vi "main002.vi"() -> ()   [LabVIEW 2018]
uses:
  subvi/Newport ESP301/Newport ESP301.lvlib
  <userlib>/caLab/Private/Put_DBL_PV.vi
  <userlib>/caLab/Private/Put_I32-1D_PV-1D.vi
  <userlib>/caLab/Private/Put_I32_PV.vi
  <userlib>/caLab/Private/Get_PV.vi
  <vilib>/DAQmx/write.llb/DAQmx Write (Analog DBL 1Chan 1Samp).vi
  <vilib>/DAQmx/create/channels.llb/DAQmx Create Channel (AO-Voltage-Basic).vi
  700a36db-ce49-4288-8972-970908bb0277.vi
  c1e43a28-daf4-4db5-b676-cc48828ec5f1.vi
panel:
  out "Intensity Graph":dbl[][](graph)
  in  "Tab Control":enum32{"Control", "Automation", "Configuration"}(tab)
  in  "delay_go":bool
  in  "delay_destination_fs":dbl=0.1 caption="Destination [fs]"
  in  "delay_destination_mm":dbl=0.1 caption="Destination [mm]"
  in  "delay_velocity":dbl=0.1 caption="velocity [mm/s]"
  in  "set_vel":bool
  in  "time_zero":dbl=1.0 caption="t0 [mm]"
  out "delay_pos_mm":dbl=1.0624 caption="Position [mm]"
  out "delay_pos_fs":dbl=416.2879908072938 caption="Time [fs]"
  in  "delay_set_t0":bool
  in  "delay_rel_mm_+":bool
  in  "delay_rel_mm_-":bool
  in  "delay_stepsize_mm":dbl=1.0 caption="step size [mm]"
  in  "delay_stepsize_fs":dbl=1.0 caption="step size [fs]"
  in  "delay_rel_fs_+":bool
  in  "delay_rel_fs_-":bool
  in  "pump_rel_+":bool
  in  "pump_rel_-":bool
  in  "pump_rel_delta":dbl=1.0 caption="step size [deg]"
  out "pump_position":dbl=1.0624 caption="Position [deg]"
  in  "probe_rel_+":bool
  in  "probe_rel_-":bool
  in  "probe_rel_delta":dbl=1.0 caption="step size [deg]"
  out "probe_position":dbl=416.2879908072938 caption="Position [deg]"
  in  "delay_mode_select":enum32{"Discrete Mode", "Continous Mode"}(tab)
  in  "delay_waypoints":string[][](table)
  in  "delay_waypoint_mode":bool=TRUE
  in  "acquisition time [ms]":u32=1000
  in  "delay_speedpoints":string[][](table)
  in  "start":bool
  in  "stop":bool
  in  "pump_waypoints":string[][](table)
  in  "pump_waypoint_mode":bool=TRUE
  in  "probe_waypoints":string[][](table)
  in  "probe_waypoint_mode":bool=TRUE
  in  "pump_offset":dbl=1.0
  in  "probe_offset":dbl=1.0
  in  "pump_set_offset":bool
  in  "probe_set_offset":bool
  in  "ESP Patch":u32[](array[numeric]) min=1 max=3 step=1
  in  "ESP301 COM PORT":refnum<visa-resource-name>="COM8"
  in  "Serial Link (RS232)":enum16{"RS232", "USB"}(ring)=enum."USB"
  in  "DAC physical channel":tag="Dev3/ao1"
  out "ESP error":errorcluster
  out "DAC error":errorcluster
  out "DAC_Voutput":dbl=5.25341140860948 caption="output voltage"
  in  "pvname_delay":string="caLabTest:DELAY"
  in  "pvname_pumprot":string="caLabTest:DELAY"
  in  "pvname_proberot":string="caLabTest:DELAY"
  in  "main_close":bool
  # "lambda / 2"
  # "Delay"
  # "lambda / 4"
  # "delaystage"
  # "stage will scan back and forth for each pump / probe angle"
  # "Pump Waveplate"
  # "Probe Waveplate"
  # "Delaystage"
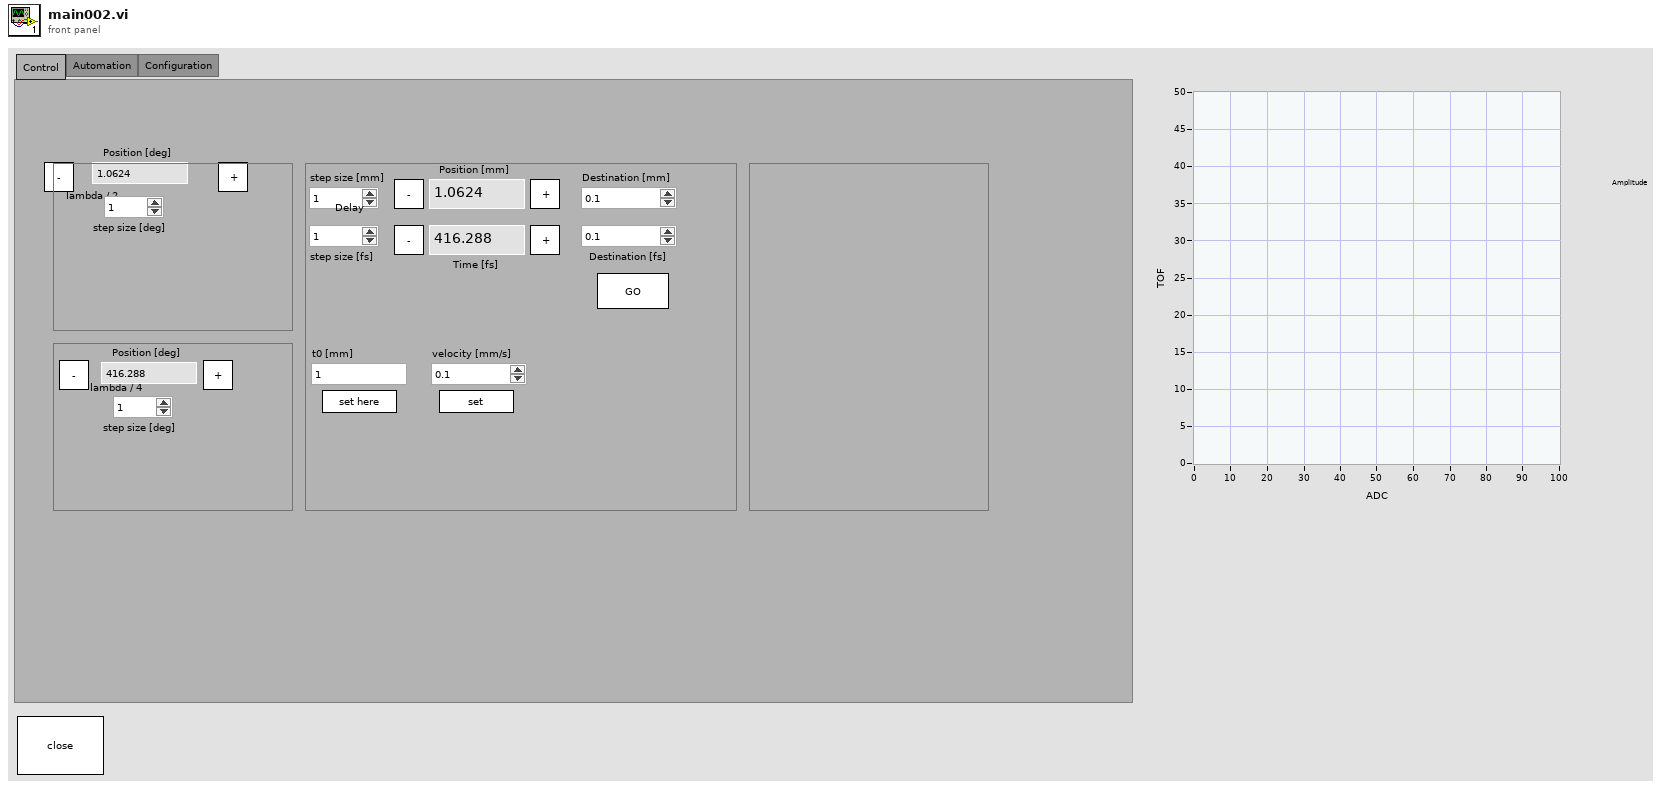
[diagram p1: front panel]
types:
  T1 = cluster{"Field Name":string, "Field Value":string}[]
  T2 = cluster{"dev1_cmd":refnum<queue>, "dev2_cmd":refnum<queue>, "meas_cmd":refnum<queue>}
  T3 = cluster{"dev1_data":refnum<queue>, "dev2_data":refnum<queue>}
  T4 = cluster{"pvname_pumprot":string, "Data Type":string, "Fields":cluster{"Field Name":string, "Field Value":string}[]}
  T5 = cluster{"pvname_delay":string, "Data Type":string, "Fields":cluster{"Field Name":string, "Field Value":string}[]}
  T6 = cluster{"pvname_proberot":string, "Data Type":string, "Fields":cluster{"Field Name":string, "Field Value":string}[]}
  T7 = cluster{"pvname_proberot":string, "Data Type":string, "Fields":cluster{"Field Name":string, "Field Value":string}[]}[]
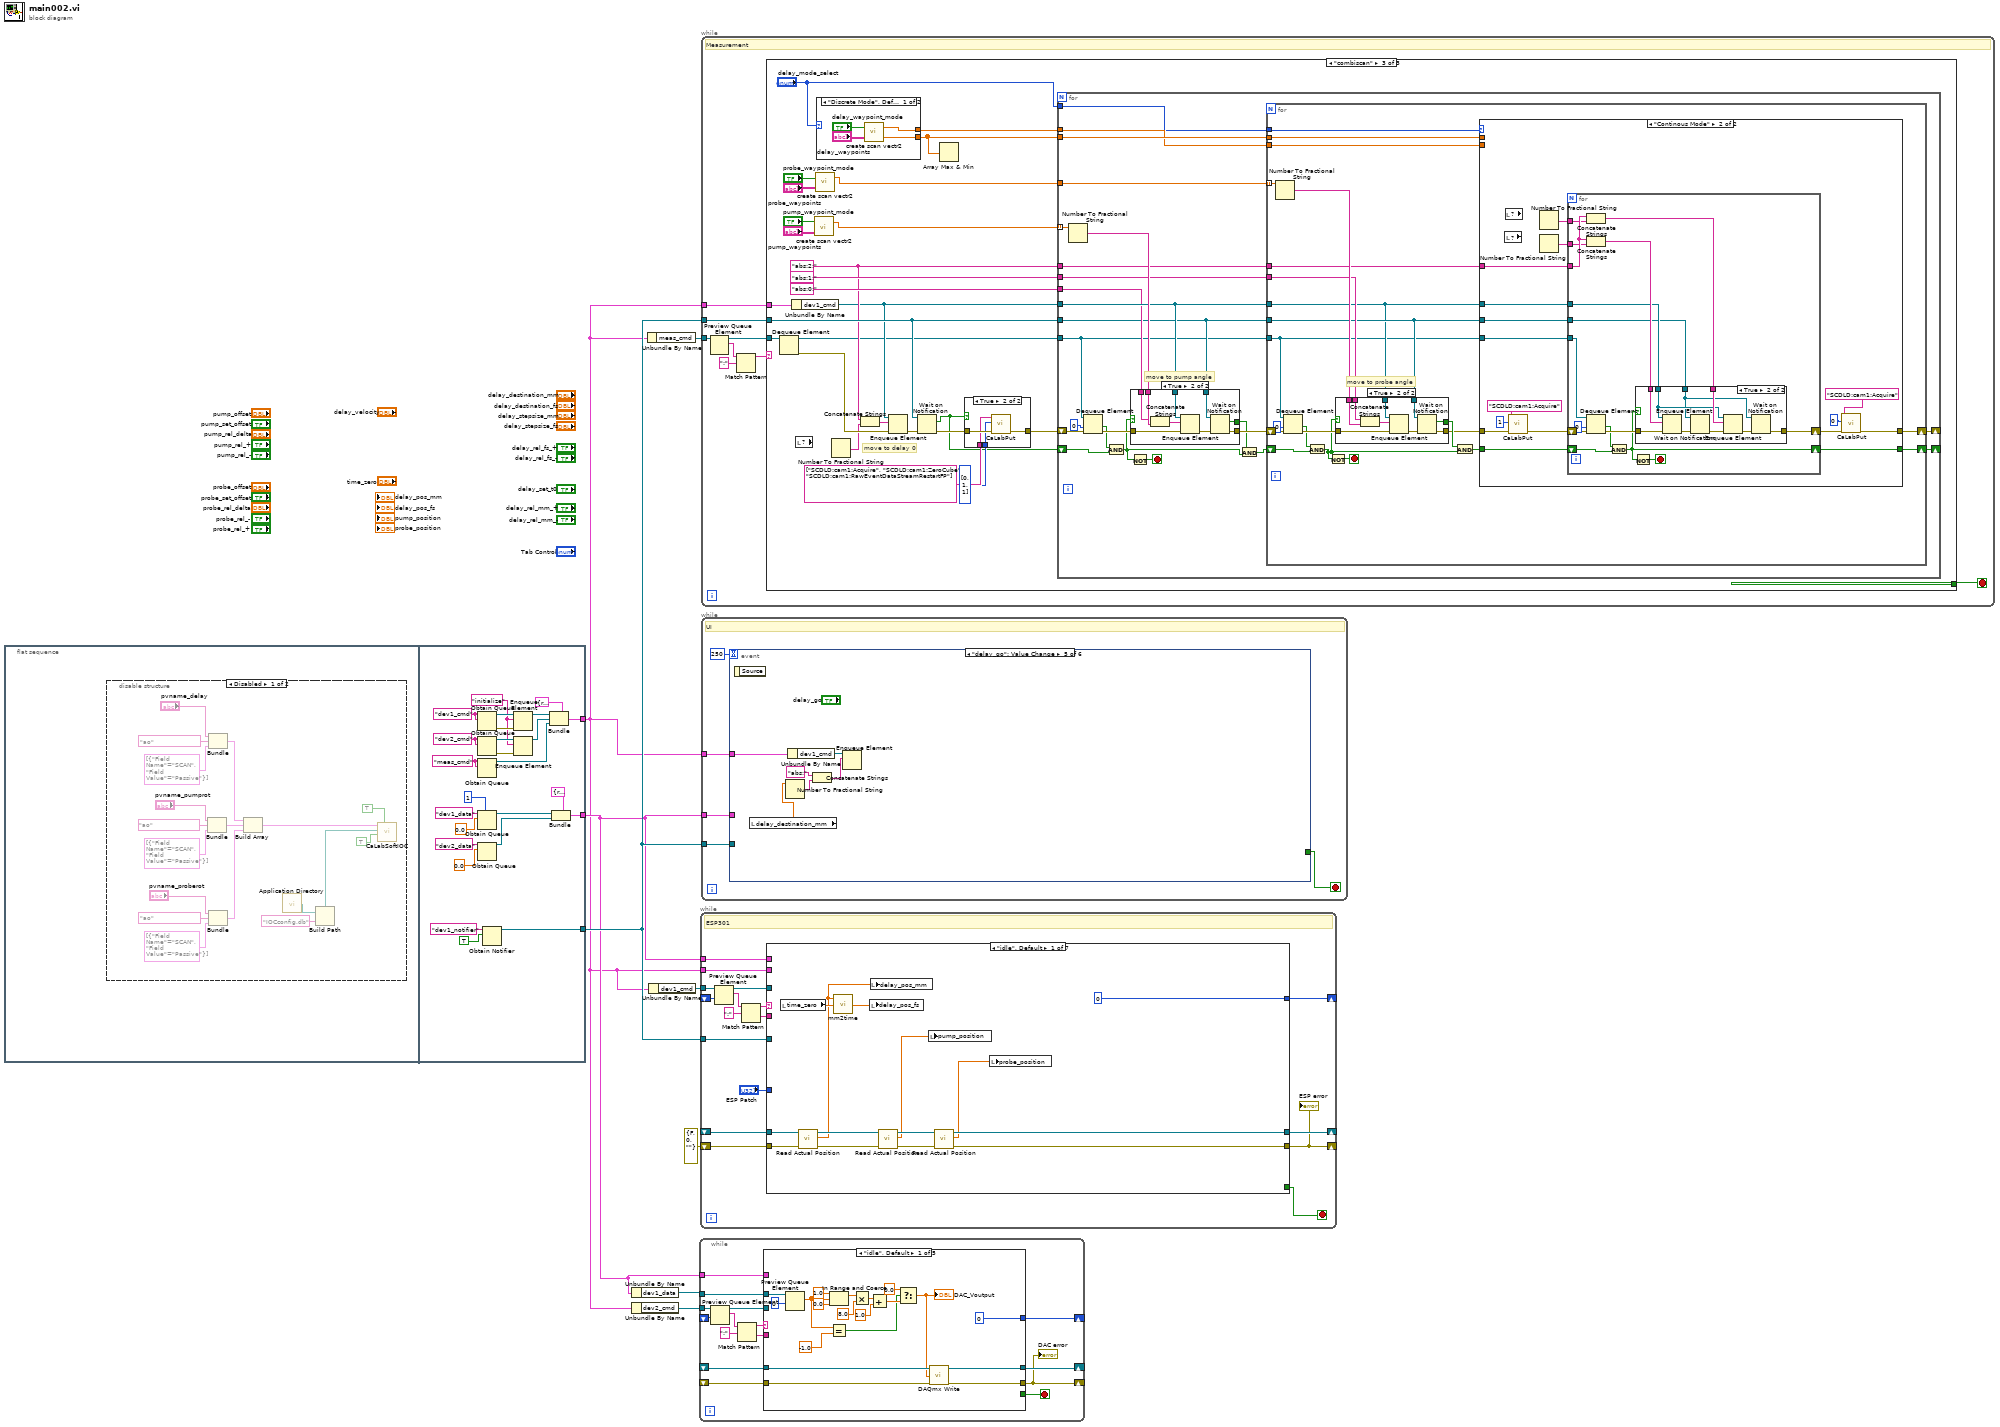
[diagram p0: block diagram]
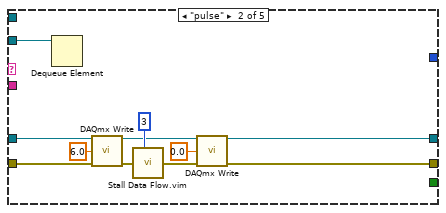
[diagram p2: hidden frame]
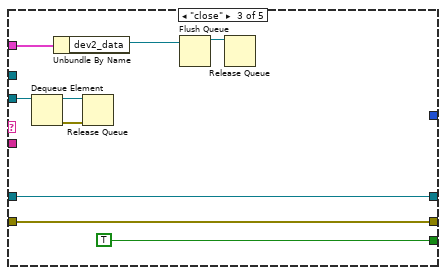
[diagram p3: hidden frame]
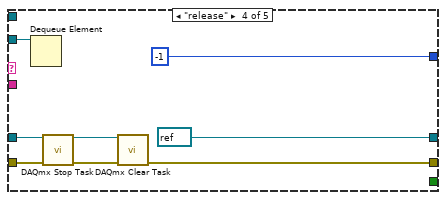
[diagram p4: hidden frame]
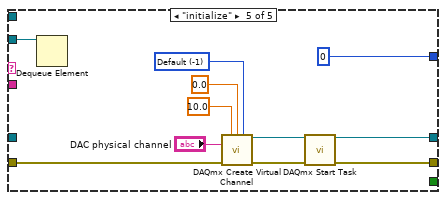
[diagram p5: hidden frame]
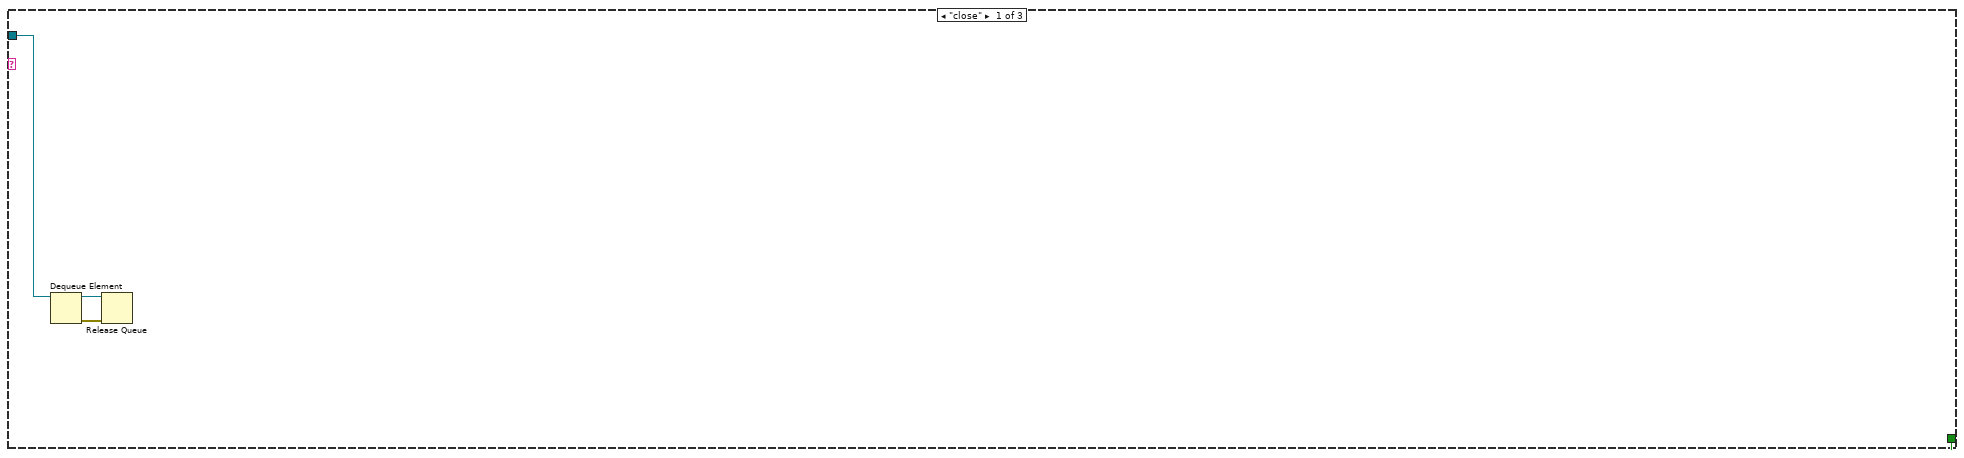
[diagram p7: hidden frame]
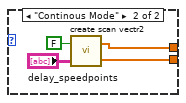
[diagram p9: hidden frame]
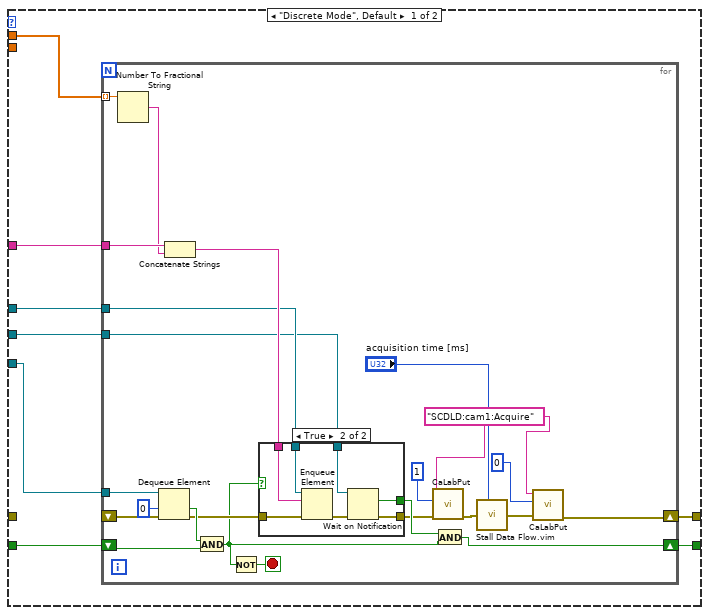
[diagram p12: hidden frame]
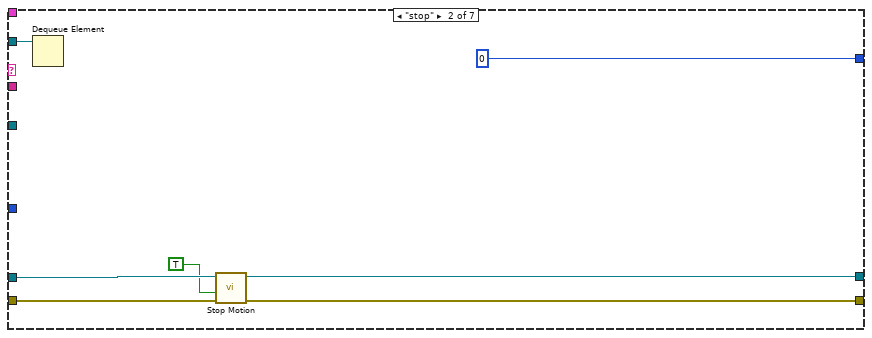
[diagram p16: hidden frame]
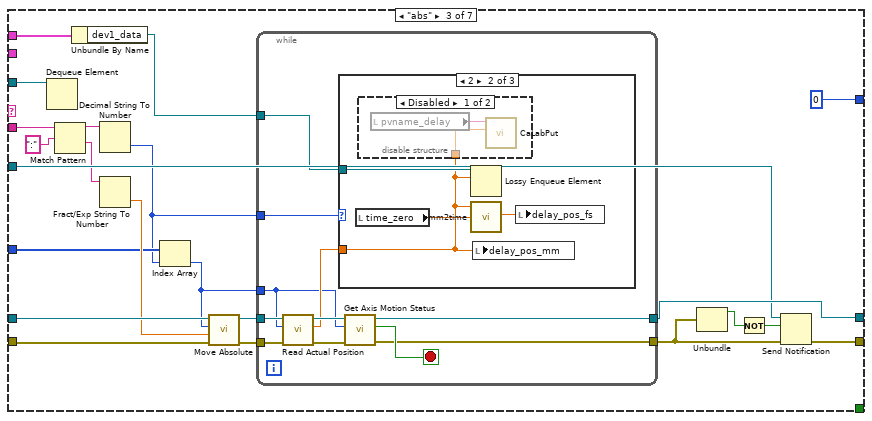
[diagram p17: hidden frame]
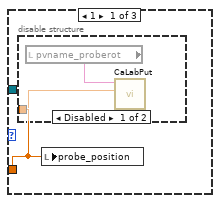
[diagram p18: hidden frame]
diagram:
  n1 = flat-sequence {
    tunnel: [w33] -> w2
    tunnel: [w28] -> w5
    tunnel: [w27] -> w1
    frame #0 {
      n2 = disable-structure shown="Disabled" {
        frame Disabled {
          n3 = Bundle("pvname_pumprot"="pvname_pumprot", "Data Type"="ao", "Fields"=T1 [{"Field Name"="SCAN", "Field Value"="Passive"}]) -> (w11:T4)  [unwired: 1 in]
          n4 = Bundle("pvname_delay"="pvname_delay", "Data Type"="ao", "Fields"=T1 [{"Field Name"="SCAN", "Field Value"="Passive"}]) -> (w18:T5)  [unwired: 1 in]
          n5 = Bundle("pvname_proberot"="pvname_proberot", "Data Type"="ao", "Fields"=T1 [{"Field Name"="SCAN", "Field Value"="Passive"}]) -> (w10:T6)  [unwired: 1 in]
          n6 = Build Array(w18, w11, w10) -> (w9:T7)
          n7 = call <vilib>:"Application Directory.vi"() -> ("Application Directory"=w25:path)
          n8 = Build Path(base path=w25, name or relative path="IOCconfig.db") -> (appended path=w26:path)
          n9 = call <userlib>:"CaLabSoftIOC.vi"("Minimize IOC"=TRUE, "Force"=TRUE, "Config File"=w26, "PV set"=w9) -> ()  [unwired: 2 in, 4 out]
        }
        frame Enabled {
        }
      }
    }
    frame #1 {
      w30 = "meas_cmd" ("name (unnamed)")
      w40 = "dev2_cmd" ("name (unnamed)")
      w45 = "initialize" ("element")
      w41 = "dev1_cmd" ("name (unnamed)")
      n10 = Obtain Queue(name (unnamed)=w41, element data type=w41) -> (queue out=w51:refnum<queue>, error out=w50:errorcluster)  [unwired: 3 in, 1 out]
      n11 = Obtain Queue(name (unnamed)=w40, element data type=w40) -> (queue out=w46:refnum<queue>, error out=w47:errorcluster)  [unwired: 3 in, 1 out]
      n12 = Obtain Queue(name (unnamed)=w30, element data type=w30) -> (queue out=w29:refnum<queue>)  [unwired: 3 in, 2 out]
      n13 = Obtain Queue(max queue size (-1, unlimited)=1, name (unnamed)="dev1_data", element data type=0.0) -> (queue out=w37:refnum<queue>)  [unwired: 2 in, 2 out]
      n14 = Obtain Queue(name (unnamed)="dev2_data", element data type=0.0) -> (queue out=w36:refnum<queue>)  [unwired: 3 in, 2 out]
      n15 = Obtain Notifier(name (unnamed)="dev1_notifier", notification data type=TRUE) -> (notifier out=w28:refnum<notifier>)  [unwired: 2 in, 2 out]
      n16 = Enqueue Element(queue=w51, element=w45, error in (no error)=w50) -> (queue out=w48:refnum<queue>)  [unwired: 1 in, 2 out]
      n17 = Enqueue Element(queue=w46, element=w45, error in (no error)=w47) -> (queue out=w44:refnum<queue>)  [unwired: 1 in, 2 out]
      n18 = Bundle(cluster=T2 {"dev1_cmd"=refnum, "dev2_cmd"=refnum, "meas_cmd"=refnum}, "dev1_cmd"=w48, "dev2_cmd"=w44, "meas_cmd"=w29) -> (w27:T2)
      n19 = Bundle(cluster=T3 {"dev1_data"=refnum, "dev2_data"=refnum}, "dev1_data"=w37, "dev2_data"=w36) -> (w33:T3)
    }
  }
  n20 = Unbundle By Name(w2) -> ("dev1_data"=w3:refnum<queue>)
  n21 = Unbundle By Name(w1) -> ("dev2_cmd"=w4:refnum<queue>)
  n22 = Unbundle By Name(w1) -> ("meas_cmd"=w6:refnum<queue>)
  n23 = Unbundle By Name(w1) -> ("dev1_cmd"=w8:refnum<queue>)
  n24 = while {
    shift-right: [w59] -> _
    shift-left: _ -> [w60]
    shift-right: [w52] -> _
    shift-left: _ -> [w58]
    tunnel: w4 -> [w57]
    shift-right: [w56] -> _
    shift-left: _ -> [w55]
    tunnel: w3 -> [w54]
    tunnel: w2 -> [w53]
    stop <- w61 stop-if-true
    n25 = Preview Queue Element(queue=w57, timeout in ms (-1)=w60) -> (queue out=w62:refnum<queue>, element=w66:string)  [unwired: 1 in, 2 out]
    n26 = Match Pattern(string=w66, regular expression=":") -> (before substring=w64:string, after substring=w63:string)  [unwired: 1 in, 2 out]
    n27 = case shown="\"idle\", Default" w64 {
      tunnel: w63 -> [_ _ _ _ _]
      tunnel: w62 -> [_ w96 w105 w112 w117]
      tunnel: [_ _ TRUE _ _] -> w61
      tunnel: [0 _ _ -1 0] -> w59
      tunnel: [w81 w86 w101 w111 w118] -> w52
      tunnel: w58 -> [w79 w88 w101 w108 w124]
      tunnel: [w82 w87 w100 refnum<k21> refnum ("task out") w119] -> w56
      tunnel: w55 -> [w80 w89 w100 w109 _]
      tunnel: w54 -> [w83 _ _ _ _]
      tunnel: w53 -> [_ _ w97 _ _]
      frame "idle", Default {
        n28 = Preview Queue Element(queue=w83, timeout in ms (-1)=0) -> (element=w72:dbl)  [unwired: 1 in, 3 out]
        n29 = In Range and Coerce(upper limit=1.0, x=w72, lower limit=0.0) -> (coerced(x)=w76:dbl)  [unwired: 1 out]
        n30 = Equal?(x=w72, y=-1.0) -> (x = y?=w68:bool)
        n31 = Multiply(x=w76, y=8.0) -> (x*y=w75:dbl)
        n32 = Add(x=w75, y=1.0 ("x")) -> (x+y=w70:dbl)
        n33 = Select(t=0.0, s=w68, f=w70) -> (s? t:f=w67:dbl)
        "DAC_Voutput" <- w67
        n34 = call-poly <vilib>:"DAQmx Write.vi"("task/channels in"=w80, "data"=w67, "error in"=w79) -> ("task out"=w82:refnum<k21>, "error out"=w81:errorcluster)  [unwired: 10 in, 1 out]
      }
      frame "pulse" {
        n35 = Dequeue Element(queue=w96) -> ()  [unwired: 2 in, 4 out]
        n36 = call-poly <vilib>:"DAQmx Write.vi"("task/channels in"=w89, "data"=6.0, "error in"=w88) -> ("task out"=w92:refnum<k21>, "error out"=w95:errorcluster)  [unwired: 10 in, 1 out]
        n37 = call "Stall Data Flow.vim"("value in"=w95, "milliseconds to wait"=u32 3) -> ("value out"=w93:errorcluster)  [unwired: 1 out]
        n38 = call-poly <vilib>:"DAQmx Write.vi"("task/channels in"=w92, "data"=0.0, "error in"=w93) -> ("task out"=w87:refnum<k21>, "error out"=w86:errorcluster)  [unwired: 10 in, 1 out]
      }
      frame "close" {
        n39 = Dequeue Element(queue=w105) -> (queue out=w104:refnum<queue>, error out=w103:errorcluster)  [unwired: 2 in, 2 out]
        n40 = Unbundle By Name(w97) -> ("dev2_data"=w98:refnum<queue>)
        n41 = Release Queue(queue=w104, error in (no error)=w103) -> ()  [unwired: 1 in, 3 out]
        n42 = Flush Queue(queue=w98) -> (queue out=w99:refnum<queue>)  [unwired: 1 in, 2 out]
        n43 = Release Queue(queue=w99) -> ()  [unwired: 2 in, 3 out]
      }
      frame "release" {
        n44 = Dequeue Element(queue=w112) -> ()  [unwired: 2 in, 4 out]
        n45 = call <vilib>:"DAQmx Stop Task.vi"("task/channels in"=w109, "error in"=w108) -> ("task out"=w107:refnum<k21>, "error out"=w106:errorcluster)  [unwired: 12 in]
        n46 = call <vilib>:"DAQmx Clear Task.vi"("task in"=w107, "error in"=w106) -> ("error out"=w111:errorcluster)  [unwired: 13 in]
      }
      frame "initialize" {
        w121 = -1 items=["Default"=-1, "RSE"=10083, "Differential"=10106, "Pseudodifferential"=12529] ("output terminal configuration")
        n47 = Dequeue Element(queue=w117) -> ()  [unwired: 2 in, 4 out]
        n48 = call-poly <vilib>:"DAQmx Create Virtual Channel.vi"("maximum value"=10.0, "minimum value"=0.0, "output terminal configuration"=w121, "physical channels"="DAC physical channel", "error in"=w124) -> ("task out"=w114:refnum<k21>, "error out"=w120:errorcluster)  [unwired: 9 in]
        n49 = call <vilib>:"DAQmx Start Task.vi"("task/channels in"=w114, "error in"=w120) -> ("task out"=w119:refnum<k21>, "error out"=w118:errorcluster)  [unwired: 12 in]
      }
    }
    "DAC error" <- w52
  }
  n50 = while {
    tunnel: w1 -> [w136]
    tunnel: w8 -> [w141]
    tunnel: w2 -> [w133]
    shift-right: [w131] -> _
    shift-left: _ -> [w132]
    shift-right: [w130] -> _
    shift-left: _ -> [w127]
    shift-right: [w129] -> _
    shift-left: errorcluster {"status"=FALSE, "code"=0, "source"=""} ("error out") -> [w128]
    tunnel: w5 -> [w126]
    stop <- w134 stop-if-true
    # "ESP301"
    n51 = Preview Queue Element(queue=w141, timeout in ms (-1)=w132) -> (queue out=w135:refnum<queue>, element=w140:string)  [unwired: 1 in, 2 out]
    n52 = Match Pattern(string=w140, regular expression=":") -> (before substring=w138:string, after substring=w137:string)  [unwired: 1 in, 2 out]
    n53 = case shown="\"idle\", Default" w138 {
      tunnel: w137 -> [_ _ w173 w211 _ _ _]
      tunnel: w136 -> [_ _ _ _ _ _ _]
      tunnel: w135 -> [_ w157 w184 w209 w225 w232 w240]
      tunnel: [_ _ _ _ TRUE _ _] -> w134
      tunnel: w133 -> [_ _ w165 _ w218 _ _]
      tunnel: [0 0 0 0 0 -1 0] -> w131
      tunnel: [w147 w160 w177 w215 w221 refnum<visa-resource-name> refnum ("VISA resource name out") w237] -> w130
      tunnel: [w146 w159 w176 w214 w220 w231 w236] -> w129
      tunnel: w128 -> [w152 w161 w182 w213 w220 w229 _]
      tunnel: w127 -> [w153 w162 w183 w212 w221 w226 _]
      tunnel: w126 -> [_ _ w175 _ _ _ _]
      tunnel: "ESP Patch" -> [_ _ w170 _ _ _ _]
      frame "idle", Default {
        n54 = local read "time_zero"() -> (w154:dbl)
        n55 = call "Read Actual Position.vi"("error in (no error)"=w152, "VISA resource name"=w153) -> ("error out"=w150:errorcluster, "Position (units)"=w144:dbl, "VISA resource name out"=w151:refnum<visa-resource-name>)  [unwired: 3 in]
        n56 = call "mm2time.vi"("Offset (mm)"=w154, "distance (mm)"=w144) -> ("time in fs"=w145:dbl)  [unwired: 1 in]
        n57 = local write "delay_pos_fs"(w145) -> ()
        n58 = local write "delay_pos_mm"(w144) -> ()
        n59 = call "Read Actual Position.vi"("error in (no error)"=w150, "VISA resource name"=w151) -> ("error out"=w148:errorcluster, "Position (units)"=w143:dbl, "VISA resource name out"=w149:refnum<visa-resource-name>)  [unwired: 3 in]
        n60 = local write "pump_position"(w143) -> ()
        n61 = call "Read Actual Position.vi"("error in (no error)"=w148, "VISA resource name"=w149) -> ("error out"=w146:errorcluster, "Position (units)"=w142:dbl, "VISA resource name out"=w147:refnum<visa-resource-name>)  [unwired: 3 in]
        n62 = local write "probe_position"(w142) -> ()
      }
      frame "stop" {
        n63 = Dequeue Element(queue=w157) -> ()  [unwired: 2 in, 4 out]
        n64 = call "Stop Motion.vi"("error in (no error)"=w161, "Stop all axes (F)"=TRUE, "VISA resource name"=w162) -> ("error out"=w159:errorcluster, "VISA resource name out"=w160:refnum<visa-resource-name>)  [unwired: 3 in]
      }
      frame "abs" {
        n65 = Dequeue Element(queue=w184) -> ()  [unwired: 2 in, 4 out]
        n66 = Match Pattern(string=w173, regular expression=":") -> (before substring=w172:string, after substring=w171:string)  [unwired: 1 in, 2 out]
        n67 = Unbundle By Name(w165) -> ("dev1_data"=w164:refnum<queue>)
        n68 = Decimal String To Number(string=w172) -> (number=w163:i32)  [unwired: 2 in, 1 out]
        n69 = Fract/Exp String To Number(string=w171) -> (number=w181:dbl)  [unwired: 3 in, 1 out]
        n70 = Index Array(array=w170, index=w163) -> (element=w169:u32)
        n71 = call "Move Absolute.vi"("error in (no error)"=w182, "Position (0 units)"=w181, "Axis (1)"=w169, "VISA resource name"=w183) -> ("error out"=w178:errorcluster, "VISA resource name out"=w179:refnum<visa-resource-name>)  [unwired: 2 in]
        n72 = while {
          tunnel: w179 -> [w195]
          tunnel: w178 -> [w194]
          tunnel: w169 -> [w187]
          tunnel: [w190] -> w177
          tunnel: [w189] -> w167
          tunnel: w164 -> [w186]
          tunnel: w163 -> [w185]
          stop <- w193 stop-if-true
          n73 = call "Read Actual Position.vi"("error in (no error)"=w194, "Axis (1)"=w187, "VISA resource name"=w195) -> ("error out"=w191:errorcluster, "Position (units)"=w188:dbl, "VISA resource name out"=w192:refnum<visa-resource-name>)  [unwired: 2 in]
          n74 = case shown="2" w185 {
            tunnel: w188 -> [w196 w199 w205]
            tunnel: w186 -> [_ w202 _]
            frame 1 {
              n75 = disable-structure shown="Disabled" {
                disable-tunnel: w196 -> [w197 _]
                frame Disabled {
                  n76 = local read "pvname_proberot"() -> (w198:string)
                  n77 = call-poly <userlib>:"CaLabPut.vi"("Value"=w197, "PV Name"=w198) -> ()  [unwired: 6 in, 4 out]
                }
                frame Enabled {
                }
              }
              n78 = local write "probe_position"(w196) -> ()
            }
            frame 2 {
              n79 = local read "time_zero"() -> (w201:dbl)
              n80 = disable-structure shown="Disabled" {
                disable-tunnel: w199 -> [w203 _]
                frame Disabled {
                  n81 = local read "pvname_delay"() -> (w204:string)
                  n82 = call-poly <userlib>:"CaLabPut.vi"("Value"=w203, "PV Name"=w204) -> ()  [unwired: 6 in, 4 out]
                }
                frame Enabled {
                }
              }
              n83 = Lossy Enqueue Element(queue=w202, element=w199) -> ()  [unwired: 1 in, 4 out]
              n84 = call "mm2time.vi"("Offset (mm)"=w201, "distance (mm)"=w199) -> ("time in fs"=w200:dbl)  [unwired: 1 in]
              n85 = local write "delay_pos_mm"(w199) -> ()
              n86 = local write "delay_pos_fs"(w200) -> ()
            }
            frame 0, Default {
              n87 = disable-structure shown="Disabled" {
                disable-tunnel: w205 -> [w207 _]
                frame Disabled {
                  n88 = local read "pvname_pumprot"() -> (w206:string)
                  n89 = call-poly <userlib>:"CaLabPut.vi"("Value"=w207, "PV Name"=w206) -> ()  [unwired: 6 in, 4 out]
                }
                frame Enabled {
                }
              }
              n90 = local write "pump_position"(w205) -> ()
            }
          }
          n91 = call "Get Axis Motion Status.vi"("error in (no error)"=w191, "Axis (1)"=w187, "VISA resource name"=w192) -> ("error out"=w189:errorcluster, "Motion Done"=w193:bool, "VISA resource name out"=w190:refnum<visa-resource-name>)  [unwired: 2 in]
        }
        n92 = Unbundle(w167) -> ("status"=w168:bool)  [unwired: 2 out]
        n93 = Not(x=w168) -> (.not. x?=w166:bool)
        n94 = Send Notification(notification=w166, notifier=w175, error in (no error)=w167) -> (error out=w176:errorcluster)  [unwired: 1 out]
      }
      frame "vel" {
        n95 = Dequeue Element(queue=w209) -> ()  [unwired: 2 in, 4 out]
        n96 = Fract/Exp String To Number(string=w211) -> (number=w210:dbl)  [unwired: 3 in, 1 out]
        n97 = call "Set Velocity.vi"("error in (no error)"=w213, "Velocity (units/s)"=w210, "VISA resource name"=w212) -> ("error out"=w214:errorcluster, "VISA resource name out"=w215:refnum<visa-resource-name>)  [unwired: 3 in]
      }
      frame "close" {
        n98 = Dequeue Element(queue=w225) -> (queue out=w224:refnum<queue>, error out=w223:errorcluster)  [unwired: 2 in, 2 out]
        n99 = Unbundle By Name(w218) -> ("dev1_data"=w216:refnum<queue>)
        n100 = Release Queue(queue=w224, error in (no error)=w223) -> ()  [unwired: 1 in, 3 out]
        n101 = Flush Queue(queue=w216) -> (queue out=w217:refnum<queue>)  [unwired: 1 in, 2 out]
        n102 = Release Queue(queue=w217) -> ()  [unwired: 2 in, 3 out]
      }
      frame "release" {
        n103 = Dequeue Element(queue=w232) -> ()  [unwired: 2 in, 4 out]
        n104 = call "Stop Motion.vi"("error in (no error)"=w229, "VISA resource name"=w226) -> ("error out"=w228:errorcluster, "VISA resource name out"=w227:refnum<visa-resource-name>)  [unwired: 4 in]
        n105 = call "Close.vi"("error in (no error)"=w228, "VISA resource name"=w227) -> ("error out"=w231:errorcluster)  [unwired: 9 in]
      }
      frame "initialize" {
        n106 = Dequeue Element(queue=w240) -> ()  [unwired: 2 in, 4 out]
        n107 = call "Initialize.vi"("VISA resource name"="ESP301 COM PORT", "error in (no error)"=errorcluster {"status"=FALSE, "code"=0, "source"=""}, "Serial Link (RS232)"="Serial Link (RS232)") -> ("VISA resource name out"=w239:refnum<visa-resource-name>, "error out"=w238:errorcluster)  [unwired: 6 in]
        n108 = call "Get Velocity.vi"("error in (no error)"=w238, "VISA resource name"=w239) -> ("error out"=w236:errorcluster, "Velocity (units/s)"=w235:dbl, "VISA resource name out"=w237:refnum<visa-resource-name>)  [unwired: 3 in]
        n109 = local write "delay_velocity"(w235) -> ()
      }
    }
    "ESP error" <- w129
  }
  n110 = while {
    tunnel: w6 -> [w249]
    tunnel: w5 -> [w244]
    tunnel: w1 -> [w245]
    stop <- w246 stop-if-true
    # "Measurement"
    n111 = Preview Queue Element(queue=w249) -> (queue out=w247:refnum<queue>, element=w250:string)  [unwired: 2 in, 2 out]
    n112 = Match Pattern(string=w250, regular expression=":") -> (before substring=w248:string)  [unwired: 1 in, 3 out]
    n113 = case shown="\"combiscan\"" w248 {
      tunnel: w247 -> [w253 _ w281]
      tunnel: [TRUE _ _] -> w246
      tunnel: w245 -> [_ _ w280]
      tunnel: w244 -> [_ _ w274]
      frame "close" {
        n114 = Dequeue Element(queue=w253) -> (queue out=w254:refnum<queue>, error out=w255:errorcluster)  [unwired: 2 in, 2 out]
        n115 = Release Queue(queue=w254, error in (no error)=w255) -> ()  [unwired: 1 in, 3 out]
      }
      frame "idle", Default {
      }
      frame "combiscan" {
        w273 = "abs:2:" ("string")
        # "move to delay 0"
        n116 = Dequeue Element(queue=w281) -> (queue out=w270:refnum<queue>, error out=w276:errorcluster)  [unwired: 2 in, 2 out]
        n117 = Unbundle By Name(w280) -> ("dev1_cmd"=w271:refnum<queue>)
        n118 = local read item#-1() -> ()  [unwired: 1 out]
        n119 = call "create scan vectr2.vi"("Table Control"="pump_waypoints", "waypoint mode?"="pump_waypoint_mode") -> ("Array"=w262:dbl[])  [unwired: 1 out]
        n120 = call "create scan vectr2.vi"("Table Control"="probe_waypoints", "waypoint mode?"="probe_waypoint_mode") -> ("Array"=w259:dbl[])  [unwired: 1 out]
        n121 = case shown="\"Discrete Mode\", Default" "delay_mode_select" {
          tunnel: [w283 w287] -> w258
          tunnel: [w282 w286] -> w256
          frame "Discrete Mode", Default {
            n122 = call "create scan vectr2.vi"("Table Control"="delay_waypoints", "waypoint mode?"="delay_waypoint_mode") -> ("Array 2"=w282:dbl[], "Array"=w283:dbl[])
          }
          frame "Continous Mode" {
            n123 = call "create scan vectr2.vi"("Table Control"="delay_speedpoints", "waypoint mode?"=FALSE) -> ("Array 2"=w286:dbl[], "Array"=w287:dbl[])
          }
        }
        n124 = Number To Fractional String() -> (F-format string=w272:string)  [unwired: 4 in]
        n125 = Concatenate Strings(w273, w272) -> (w277:string)
        n126 = Enqueue Element(queue=w271, element=w277, error in (no error)=w276) -> (error out=w275:errorcluster)  [unwired: 1 in, 2 out]
        n127 = Wait on Notification(notifier=w274, error in (no error)=w275) -> (notification=w265:bool, error out=w269:errorcluster)  [unwired: 2 in, 2 out]
        n128 = Array Max & Min(array=w256) -> ()  [unwired: 4 out]
        n129 = case shown="True" w265 {
          tunnel: w269 -> [w290 w294]
          tunnel: string[] ["SCDLD:cam1:Acquire", "SCDLD:cam1:ZeroCube", "SCDLD:cam1:RawEventDataStreamRestartFP"] ("PV Names") -> [_ w293]
          tunnel: i32[] [0, 1, 1] -> [_ w292]
          tunnel: [w290 w291] -> w266
          frame False {
          }
          frame True {
            n130 = call-poly <userlib>:"CaLabPut.vi"("Error in (no error)"=w294, "Values"=w292, "PV Names"=w293) -> ("Error out"=w291:errorcluster)  [unwired: 5 in, 3 out]
          }
        }
        n131 = for {
          tunnel: w262 -> [w317] mode=indexing
          tunnel: w259 -> [w318]
          tunnel: w274 -> [w311]
          tunnel: w271 -> [w315]
          tunnel: "abs:0:" ("string") -> [w314]
          tunnel: "abs:1:" ("string") -> [w313]
          tunnel: w273 -> [w310]
          tunnel: w270 -> [w307]
          shift-right: [w303] -> _
          shift-left: w265 -> [w304]
          shift-right: [w301] -> _
          shift-left: w266 -> [w309]
          tunnel: w258 -> [w300]
          tunnel: "delay_mode_select" -> [w296]
          tunnel: w256 -> [w295]
          stop <- w302 stop-if-true
          # "move to pump angle"
          n132 = Number To Fractional String(number=w317) -> (F-format string=w316:string)  [unwired: 3 in]
          n133 = Dequeue Element(queue=w307, timeout in ms (-1)=0, error in (no error)=w309) -> (timed out?=w305:bool, error out=w308:errorcluster)  [unwired: 2 out]
          n134 = And(x=w305, y=w304) -> (x .and. y?=w299:bool)
          n135 = case shown="True" w299 {
            selector: w299 -> [w319 _]
            tunnel: w316 -> [_ w329]
            tunnel: w315 -> [_ w327]
            tunnel: w314 -> [_ w326]
            tunnel: [w320 w324] -> w312
            tunnel: w311 -> [_ w323]
            tunnel: w308 -> [w320 w322]
            tunnel: [w319 w321] -> w298
            frame False {
            }
            frame True {
              n136 = Concatenate Strings(w326, w329) -> (w328:string)
              n137 = Enqueue Element(queue=w327, element=w328, error in (no error)=w322) -> (error out=w325:errorcluster)  [unwired: 1 in, 2 out]
              n138 = Wait on Notification(notifier=w323, error in (no error)=w325) -> (notification=w321:bool, error out=w324:errorcluster)  [unwired: 2 in, 2 out]
            }
          }
          n139 = Not(x=w299) -> (.not. x?=w302:bool)
          n140 = And(x=w298, y=w299) -> (x .and. y?=w297:bool)
          n141 = for {
            tunnel: w318 -> [w351] mode=indexing
            tunnel: w311 -> [w348]
            tunnel: w315 -> [w346]
            tunnel: w313 -> [w349]
            tunnel: w310 -> [w347]
            tunnel: w307 -> [w343]
            shift-right: [w339] -> w303
            shift-left: w297 -> [w341]
            shift-right: [w331] -> w301
            shift-left: w312 -> [w345]
            tunnel: w300 -> [w337]
            tunnel: w296 -> [w333]
            tunnel: w295 -> [w330]
            stop <- w340 stop-if-true
            # "move to probe angle"
            n142 = Number To Fractional String(number=w351) -> (F-format string=w350:string)  [unwired: 3 in]
            n143 = Dequeue Element(queue=w343, timeout in ms (-1)=0, error in (no error)=w345) -> (timed out?=w342:bool, error out=w344:errorcluster)  [unwired: 2 out]
            n144 = And(x=w342, y=w341) -> (x .and. y?=w335:bool)
            n145 = Not(x=w335) -> (.not. x?=w340:bool)
            n146 = case shown="True" w335 {
              selector: w335 -> [w435 _]
              tunnel: w350 -> [_ w444]
              tunnel: w349 -> [_ w443]
              tunnel: w348 -> [_ w441]
              tunnel: [w436 w440] -> w332
              tunnel: w346 -> [_ w439]
              tunnel: w344 -> [w436 w438]
              tunnel: [w435 w437] -> w336
              frame False {
              }
              frame True {
                n147 = Concatenate Strings(w443, w444) -> (w445:string)
                n148 = Enqueue Element(queue=w439, element=w445, error in (no error)=w438) -> (error out=w442:errorcluster)  [unwired: 1 in, 2 out]
                n149 = Wait on Notification(notifier=w441, error in (no error)=w442) -> (notification=w437:bool, error out=w440:errorcluster)  [unwired: 2 in, 2 out]
              }
            }
            n150 = And(x=w336, y=w335) -> (x .and. y?=w334:bool)
            n151 = case shown="\"Continous Mode\"" w333 {
              tunnel: w348 -> [w352 w408]
              tunnel: w347 -> [w354 w407]
              tunnel: w346 -> [w353 w406]
              tunnel: w343 -> [w355 w405]
              tunnel: w334 -> [w359 w402]
              tunnel: [w357 w401] -> w339
              tunnel: [w358 w393] -> w331
              tunnel: w337 -> [w356 _]
              tunnel: w332 -> [_ w400]
              tunnel: w330 -> [_ _]
              frame "Discrete Mode", Default {
                n152 = for {
                  shift-right: [w368] -> w357
                  shift-left: w359 -> [w378]
                  shift-right: [w365] -> w358
                  shift-left: _ -> [w380]
                  tunnel: w356 -> [w376] mode=indexing
                  tunnel: w355 -> [w379]
                  tunnel: w354 -> [w375]
                  tunnel: w353 -> [w372]
                  tunnel: w352 -> [w371]
                  stop <- w383 stop-if-true
                  w364 = "SCDLD:cam1:Acquire"
                  n153 = Number To Fractional String(number=w376) -> (F-format string=w374:string)  [unwired: 3 in]
                  n154 = Dequeue Element(queue=w379, timeout in ms (-1)=0, error in (no error)=w380) -> (timed out?=w382:bool, error out=w377:errorcluster)  [unwired: 2 out]
                  n155 = Concatenate Strings(w375, w374) -> (w373:string)
                  n156 = And(x=w382, y=w378) -> (x .and. y?=w370:bool)
                  n157 = Not(x=w370) -> (.not. x?=w383:bool)
                  n158 = case shown="True" w370 {
                    selector: w370 -> [w384 _]
                    tunnel: w377 -> [w385 w391]
                    tunnel: [w385 w390] -> w366
                    tunnel: w373 -> [_ w389]
                    tunnel: w372 -> [_ w388]
                    tunnel: w371 -> [_ w387]
                    tunnel: [w384 w386] -> w369
                    frame False {
                    }
                    frame True {
                      n159 = Enqueue Element(queue=w388, element=w389, error in (no error)=w391) -> (error out=w392:errorcluster)  [unwired: 1 in, 2 out]
                      n160 = Wait on Notification(notifier=w387, error in (no error)=w392) -> (notification=w386:bool, error out=w390:errorcluster)  [unwired: 2 in, 2 out]
                    }
                  }
                  n161 = call-poly <userlib>:"CaLabPut.vi"("Error in (no error)"=w366, "Value"=1, "PV Name"=w364) -> ("Error out"=w362:errorcluster)  [unwired: 5 in, 3 out]
                  n162 = And(x=w369, y=w370) -> (x .and. y?=w368:bool)
                  n163 = call "Stall Data Flow.vim"("value in"=w362, "milliseconds to wait"="acquisition time [ms]") -> ("value out"=w361:errorcluster)  [unwired: 1 out]
                  n164 = call-poly <userlib>:"CaLabPut.vi"("Error in (no error)"=w361, "Value"=0, "PV Name"=w364) -> ("Error out"=w365:errorcluster)  [unwired: 5 in, 3 out]
                }
              }
              frame "Continous Mode" {
                n165 = local read item#-1() -> ()  [unwired: 1 out]
                n166 = local read item#-1() -> ()  [unwired: 1 out]
                n167 = call-poly <userlib>:"CaLabPut.vi"("Error in (no error)"=w400, "Value"=1, "PV Name"="SCDLD:cam1:Acquire") -> ("Error out"=w397:errorcluster)  [unwired: 5 in, 3 out]
                n168 = Number To Fractional String() -> (F-format string=w403:string)  [unwired: 4 in]
                n169 = Number To Fractional String() -> (F-format string=w404:string)  [unwired: 4 in]
                n170 = for {
                  tunnel: w408 -> [w420]
                  tunnel: w407 -> [w422]
                  tunnel: w406 -> [w421]
                  tunnel: w405 -> [w417]
                  shift-right: [w412] -> w401
                  shift-left: w402 -> [w414]
                  tunnel: w404 -> [w416]
                  tunnel: w403 -> [w415]
                  shift-right: [w410] -> w394
                  shift-left: w397 -> [w419]
                  stop <- w411 stop-if-true
                  n171 = Concatenate Strings(w422, w416) -> (w423:string)
                  n172 = Concatenate Strings(w422, w415) -> (w424:string)
                  n173 = Dequeue Element(queue=w417, timeout in ms (-1)=0, error in (no error)=w419) -> (timed out?=w413:bool, error out=w418:errorcluster)  [unwired: 2 out]
                  n174 = And(x=w413, y=w414) -> (x .and. y?=w412:bool)
                  n175 = Not(x=w412) -> (.not. x?=w411:bool)
                  n176 = case shown="True" w412 {
                    tunnel: w424 -> [_ w433]
                    tunnel: w423 -> [_ w432]
                    tunnel: w421 -> [_ w429]
                    tunnel: w420 -> [_ w428]
                    tunnel: w418 -> [w425 w427]
                    tunnel: [w425 w426] -> w410
                    frame False {
                    }
                    frame True {
                      n177 = Enqueue Element(queue=w429, element=w433, error in (no error)=w427) -> (error out=w434:errorcluster)  [unwired: 1 in, 2 out]
                      n178 = Wait on Notification(notifier=w428, error in (no error)=w434) -> (error out=w430:errorcluster)  [unwired: 2 in, 3 out]
                      n179 = Enqueue Element(queue=w429, element=w432, error in (no error)=w430) -> (error out=w431:errorcluster)  [unwired: 1 in, 2 out]
                      n180 = Wait on Notification(notifier=w428, error in (no error)=w431) -> (error out=w426:errorcluster)  [unwired: 2 in, 3 out]
                    }
                  }
                }
                n181 = call-poly <userlib>:"CaLabPut.vi"("Error in (no error)"=w394, "Value"=0, "PV Name"="SCDLD:cam1:Acquire") -> ("Error out"=w393:errorcluster)  [unwired: 5 in, 3 out]
              }
            }
          }
        }
      }
    }
  }
  n182 = while {
    tunnel: w1 -> [w450]
    tunnel: w2 -> [w449]
    tunnel: w5 -> [w447]
    stop <- w448 stop-if-true
    # "UI"
    n183 = event shown="[4] \"delay_go\": Value Change" {
      selector: _ -> [_ _ _ _ _ _]
      dyn-events: _ -> [_ _ _ _ _ _]
      timeout: 250 -> [_ _ _ _ _ _]
      tunnel: w450 -> [_ w459 w464 w467 w477 w480]
      tunnel: w449 -> [_ _ _ _ _ _]
      tunnel: [_ _ _ _ _ TRUE] -> w448
      tunnel: w447 -> [_ _ _ _ _ _]
      event Timeout {
        n184 = event-data() -> ()  [unwired: 1 in, 1 out]
        n185 = call-poly <userlib>:"CaLabGet.vi"("PV Name"="SCDLD:CPProjectionData_History_P0_2D:ArrayData") -> ("Value Array (number)"=w456:dbl[])  [unwired: 8 in, 6 out]
        n186 = call-poly <userlib>:"CaLabGet.vi"("PV Name"="SCDLD:cam1:CPSize_P1_2D_A1") -> ("1rst Value (number)"=w453:dbl)  [unwired: 8 in, 6 out]
        n187 = call-poly <userlib>:"CaLabGet.vi"("PV Name"="SCDLD:cam1:CPSize_P1_2D_A0") -> ("1rst Value (number)"=w452:dbl)  [unwired: 8 in, 6 out]
        n188 = Reshape Array(w456, w453, w452) -> (→"Intensity Graph":dbl[][])
      }
      event "start": Value Change {
        n189 = event-data() -> ()  [unwired: 1 in, 1 out]
        n190 = Unbundle By Name(w459) -> ("meas_cmd"=w460:refnum<queue>)
        n191 = Enqueue Element(queue=w460, element="combiscan" ("string")) -> ()  [unwired: 2 in, 3 out]
      }
      event "stop": Value Change {
        n192 = event-data() -> ()  [unwired: 1 in, 1 out]
        n193 = Unbundle By Name(w464) -> ("meas_cmd"=w463:refnum<queue>)
        n194 = Flush Queue(queue=w463) -> (queue out=w462:refnum<queue>, error out=w461:errorcluster)  [unwired: 1 in, 1 out]
        n195 = Enqueue Element(queue=w462, element="stop" ("string"), error in (no error)=w461) -> ()  [unwired: 1 in, 3 out]
      }
      event "set_vel": Value Change {
        n196 = event-data() -> ()  [unwired: 1 in, 2 out]
        n197 = local read "delay_velocity"() -> (w466:dbl)
        n198 = Number To Fractional String(number=w466) -> (F-format string=w470:string)  [unwired: 3 in]
        n199 = Unbundle By Name(w467) -> ("dev1_cmd"=w471:refnum<queue>)
        n200 = Concatenate Strings("vel:" ("string"), w470) -> (w469:string)
        n201 = Enqueue Element(queue=w471, element=w469) -> ()  [unwired: 2 in, 3 out]
      }
      event "delay_go": Value Change {
        n202 = event-data() -> ()  [unwired: 1 in, 1 out]
        n203 = local read "delay_destination_mm"() -> (w472:dbl)
        n204 = Number To Fractional String(number=w472) -> (F-format string=w475:string)  [unwired: 3 in]
        n205 = Unbundle By Name(w477) -> ("dev1_cmd"=w476:refnum<queue>)
        n206 = Concatenate Strings("abs:" ("string"), w475) -> (w473:string)
        n207 = Enqueue Element(queue=w476, element=w473) -> ()  [unwired: 2 in, 3 out]
      }
      event "main_close": Value Change {
        n208 = event-data() -> ()  [unwired: 1 in, 1 out]
        n209 = Cluster To Array(cluster=w480) -> (array=w479:refnum<queue>[])
        n210 = for {
          tunnel: w479 -> [w485] mode=indexing
          n211 = Flush Queue(queue=w485) -> (queue out=w481:refnum<queue>)  [unwired: 1 in, 2 out]
          n212 = Enqueue Element(queue=w481, element="release") -> (queue out=w483:refnum<queue>)  [unwired: 2 in, 2 out]
          n213 = Enqueue Element(queue=w483, element="close") -> ()  [unwired: 2 in, 3 out]
        }
      }
    }
  }
